vi "Read Message.vi"(8 "error in (no error)":errorcluster, 9 "Timeout mS (-1)":i32=-1, 11 "Actor API in":refnum<class "Actor API.lvclass">) -> (0 "error out":errorcluster, 1 "Timeout":bool, 2 "Message":refnum<class "Message.lvclass">, 3 "Actor API out":refnum<class "Actor API.lvclass">)   [LabVIEW 2022 SP3, in "Artifex.lvlib" / "Actor API.lvclass"]
uses:
  Actor API.lvclass
  Message/Message.lvclass
  Actor API.lvclass/Actor API.ctl
  Priority Message Queue/Priority Message Queue.lvclass
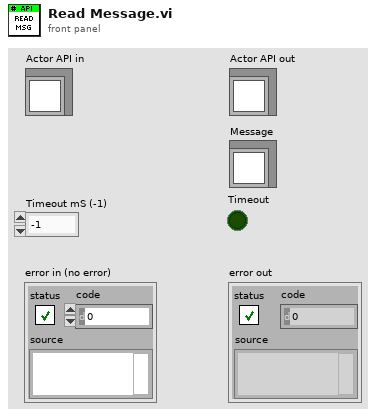
[diagram p1: front panel]
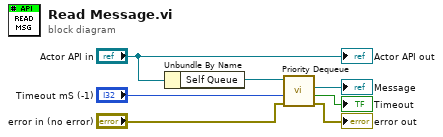
[diagram p0: block diagram]
diagram:
  n1 = Unbundle By Name("Actor API in") -> ("Self Queue"=w6:refnum<class "Priority Message Queue.lvclass">)
  n2 = call "Priority Dequeue.vi"("error in (no error)"="error in (no error)", "Timeout mS (-1)"="Timeout mS (-1)", "Priority Message Queue in"=w6) -> ("error out"=→"error out":errorcluster, "Timed Out"=→"Timeout":bool, "Message"=→"Message":refnum<class "Message.lvclass">)  [unwired: 4 in, 2 out]
  "Actor API out" <- "Actor API in"
